vi "EnFlo_Data_Sync_Manual.vi"() -> ()   [LabVIEW 2015]
uses:
  Anemometry Sub Vis/Controls/EnFlo_Data_Folder_Setup.ctl
  ADAM Client/Sub VIs/Harvest_Global.vi
  Anemometry Sub Vis/Globals/Preference_global.vi
  Anemometry Sub Vis/Globals/Constants_global.vi
panel:
  in  "Age in Days of files":dbl=nan
  out "Files Copied fr Local to Public":i32
  out "Files pulled from Public":i32
  in  "stop":bool
  out "Files Copied fr Server to Public":i32
  out "No Files to Push":i32
  out "No of Files to Pull":i32
  out "Files pushed onto Server":i32
  out "File being transfered":path
  out "Currently":string
  out "Files to Pull From Server":path[](array[path])
  out "Files to Push to Server":path[](array[path])
  in  "Browse Remote Disk":bool
  out "error out":errorcluster
  out "Folder contents changed?":bool
  in  "Folder to Sync (Must be within Local EnFlo Data)":path=path "C:/EnFlo_Data_Temp/EnFlo_Software_SVN"
  in  "Get all Server Files":bool=TRUE
  in  "Check Updates on Server?":bool=TRUE
  in  "Archive Files?":bool
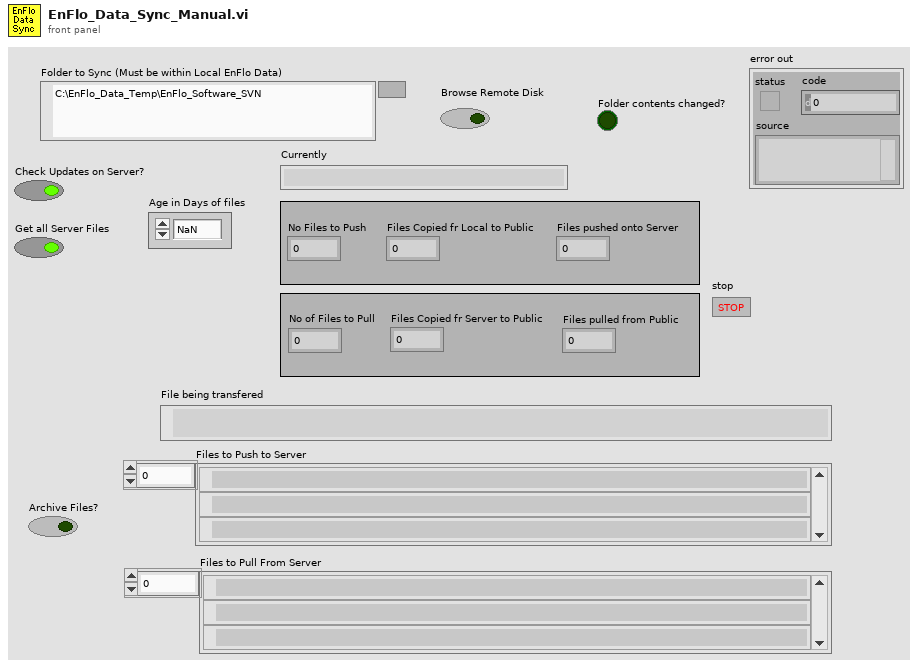
[diagram p1: front panel]
types:
  T1 = typedef "EnFlo_Data_Folder_Setup.ctl" = string
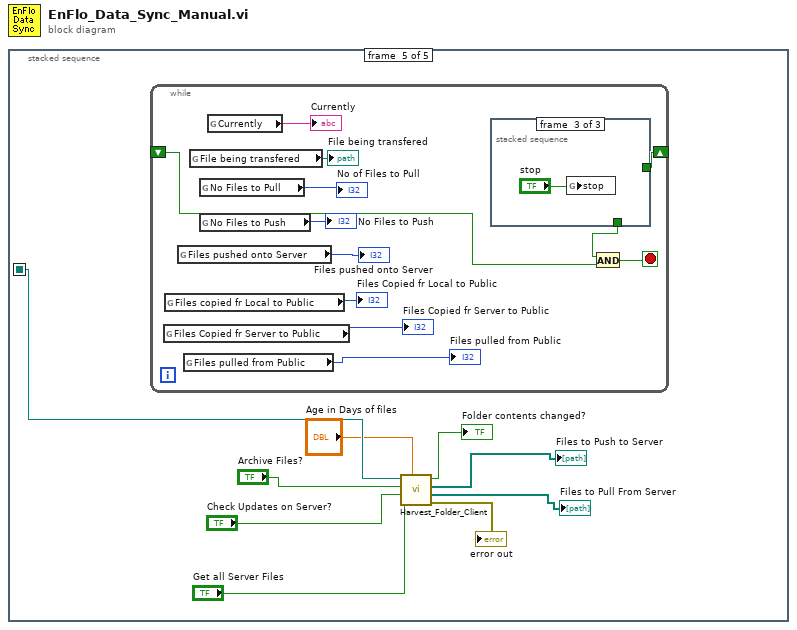
[diagram p0: block diagram]
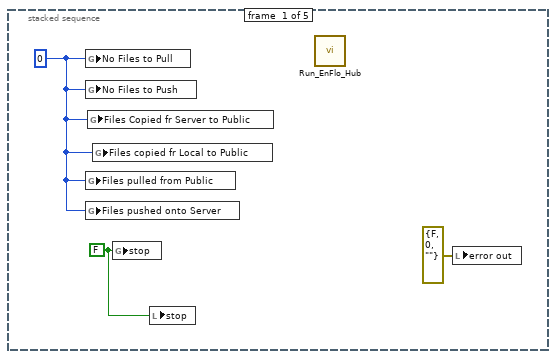
[diagram p2: hidden frame]
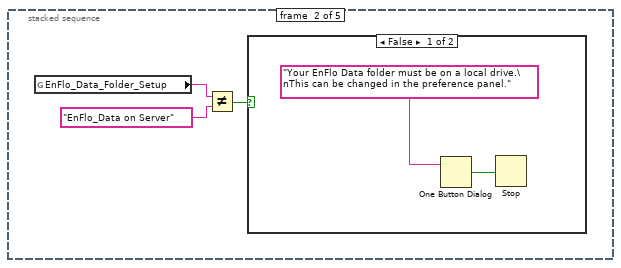
[diagram p3: hidden frame]
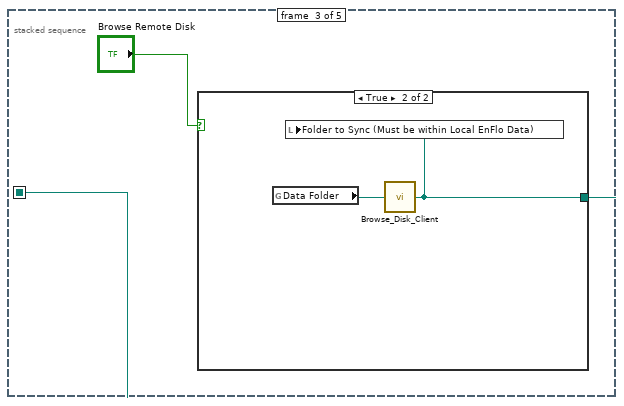
[diagram p5: hidden frame]
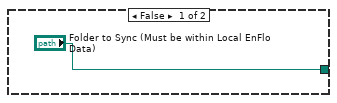
[diagram p6: hidden frame]
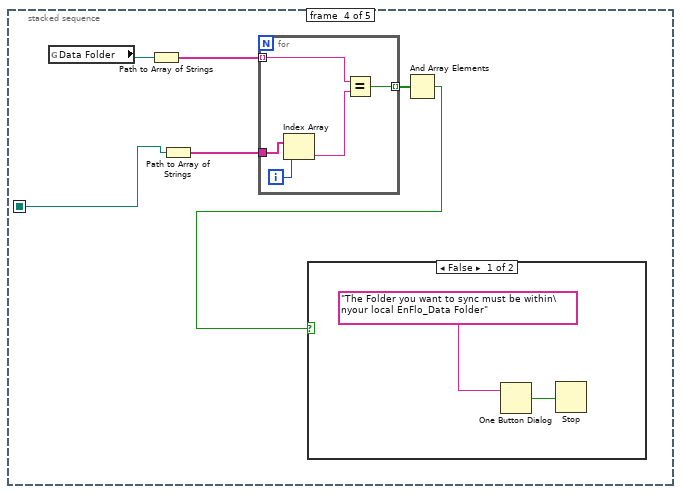
[diagram p7: hidden frame]
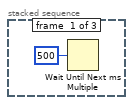
[diagram p9: hidden frame]
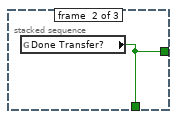
[diagram p10: hidden frame]
diagram:
  n1 = stacked-sequence {
    seq-local: [_ _ w9 _ _] -> [_ _ _ w14 w31]
    frame #0 {
      w2 = FALSE ("stop")
      w3 = 0 ("No Files to Pull")
      n2 = global write "Harvest_Global.vi" "No Files to Pull"(w3) -> ()
      n3 = global write "Harvest_Global.vi" "No Files to Push"(w3) -> ()
      n4 = global write "Harvest_Global.vi" "Files pulled from Public"(w3) -> ()
      n5 = global write "Harvest_Global.vi" "Files pushed onto Server"(w3) -> ()
      n6 = global write "Harvest_Global.vi" "Files Copied fr Server to Public"(w3) -> ()
      n7 = global write "Harvest_Global.vi" "Files copied fr Local to Public"(w3) -> ()
      n8 = global write "Harvest_Global.vi" "stop"(w2) -> ()
      n9 = local write "stop"(w2) -> ()
      n10 = call "Run_EnFlo_Hub.vi"() -> ()  [unwired: 8 in]
      n11 = local write "error out"(errorcluster {"status"=FALSE, "code"=0, "source"=""} ("error out")) -> ()
    }
    frame #1 {
      n12 = global read "Preference_global.vi" "EnFlo_Data_Folder_Setup"() -> (w5:T1)
      n13 = Not Equal?(x=w5, y=T1 "EnFlo_Data on Server" ("EnFlo_Data_Folder_Setup")) -> (x != y?=w6:bool)
      n14 = case shown="False" w6 {
        frame False {
          n15 = One Button Dialog(message="Your EnFlo Data folder must be on a local drive.\nThis can be changed in the preference panel.") -> (true=w7:bool)  [unwired: 1 in]
          n16 = Stop(stop? (T)=w7) -> ()
        }
        frame True {
        }
      }
    }
    frame #2 {
      n17 = case shown="True" "Browse Remote Disk" {
        tunnel: ["Folder to Sync (Must be within Local EnFlo Data)" w12] -> w9
        frame False {
        }
        frame True {
          n18 = global read "Constants_global.vi" "Data Folder"() -> (w13:path)
          n19 = call "Browse_Disk_Client.vi"("Start Path"=w13) -> ("Folder to Pull from Server"=w12:path)
          n20 = local write "Folder to Sync (Must be within Local EnFlo Data)"(w12) -> ()
        }
      }
    }
    frame #3 {
      n21 = global read "Constants_global.vi" "Data Folder"() -> (w19:path)
      n22 = Path to Array of Strings(0:w19) -> (2:w17:string[])  [unwired: 1 out]
      n23 = Path to Array of Strings(0:w14) -> (2:w18:string[])  [unwired: 1 out]
      n24 = for {
        tunnel: w18 -> [w24]
        tunnel: w17 -> [w22] mode=indexing
        tunnel: [w20] -> w16 mode=indexing
        i -> [w23]
        n25 = Index Array(array=w24, index=w23) -> (element=w21:string)
        n26 = Equal?(x=w22, y=w21) -> (x = y?=w20:bool)
      }
      n27 = And Array Elements(Boolean array=w16) -> (logical AND=w15:bool)
      n28 = case shown="False" w15 {
        frame False {
          n29 = One Button Dialog(message="The Folder you want to sync must be within\nyour local EnFlo_Data Folder") -> (true=w25:bool)  [unwired: 1 in]
          n30 = Stop(stop? (T)=w25) -> ()
        }
        frame True {
        }
      }
    }
    frame #4 {
      n31 = while {
        shift-right: [w43] -> _
        shift-left: _ -> [w40]
        stop <- w42 stop-if-true
        n32 = global read "Harvest_Global.vi" "Files Copied fr Server to Public"() -> (→"Files Copied fr Server to Public":i32)
        n33 = global read "Harvest_Global.vi" "Files copied fr Local to Public"() -> (→"Files Copied fr Local to Public":i32)
        n34 = global read "Harvest_Global.vi" "Files pushed onto Server"() -> (→"Files pushed onto Server":i32)
        n35 = global read "Harvest_Global.vi" "Files pulled from Public"() -> (→"Files pulled from Public":i32)
        n36 = global read "Harvest_Global.vi" "File being transfered"() -> (→"File being transfered":path)
        n37 = global read "Harvest_Global.vi" "No Files to Pull"() -> (→"No of Files to Pull":i32)
        n38 = global read "Harvest_Global.vi" "No Files to Push"() -> (→"No Files to Push":i32)
        n39 = global read "Harvest_Global.vi" "Currently"() -> (→"Currently":string)
        n40 = stacked-sequence {
          tunnel: [_ w49 _] -> w41
          tunnel: [_ w49 _] -> w43
          frame #0 {
            n41 = Wait Until Next ms Multiple(millisecond multiple=u32 500) -> ()  [unwired: 1 out]
          }
          frame #1 {
            n42 = global read "Harvest_Global.vi" "Done Transfer?"() -> (w49:bool)
          }
          frame #2 {
            n43 = global write "Harvest_Global.vi" "stop"("stop") -> ()
          }
        }
        n44 = And(x=w41, y=w40) -> (x .and. y?=w42:bool)
      }
      n45 = call "Harvest_Folder_Client.vi"("Age in Days of files"="Age in Days of files", "Get all Server Files"="Get all Server Files", "Check Updates on Server?"="Check Updates on Server?", "Archive Files?"="Archive Files?", "Folder to Harvest"=w31) -> ("error out"=→"error out":errorcluster, "Files to Pull From Server"=→"Files to Pull From Server":path[], "Files to Push to Server"=→"Files to Push to Server":path[], "Folder contents changed?"=→"Folder contents changed?":bool)
    }
  }
